vi "Write Serialized Configuration Parameter.vi"(8 "error in (no error)":errorcluster, 10 "Serialized Configuration":string, 11 "RandomNumberLogger in":refnum<class "RandomNumberLogger.lvclass">) -> (0 "error out":errorcluster, 3 "RandomNumberLogger out":refnum<class "RandomNumberLogger.lvclass">)   [LabVIEW 2020, in "RandomNumberLogger.lvlib" / "RandomNumberLogger.lvclass"]
doc: "<b>Write Serialized Configuration Parameter</b>\nThis method writes the serialized configuration data to th class data in the plugin."
uses:
  RandomNumberLogger.lvclass
  C:/Program Files/National Instruments/LabVIEW 2020/vi.lib/FlexLogger/SDK/PluginSDK.lvlibp/PEFClasses/SDK/Processing Element/Processing Element.lvclass
  <vilib>/FlexLogger/SDK/PluginSDK.lvlibp/PEFClasses/SDK/Processing Element/Read Parameters Property.vi
  <vilib>/FlexLogger/SDK/PluginSDK.lvlibp/PEFClasses/SDK/Parameters/SetParameter(String).vi
  <vilib>/FlexLogger/SDK/PluginSDK.lvlibp/PEFClasses/SDK/Processing Element/Write Parameters Property.vi
  <vilib>/FlexLogger/SDK/PluginSDK.lvlibp/PEFClasses/SDK/Parameters/Parameters.lvclass
  RandomNumberLogger.lvclass/RandomNumberLogger.ctl
panel:
  # "#via_ignore"
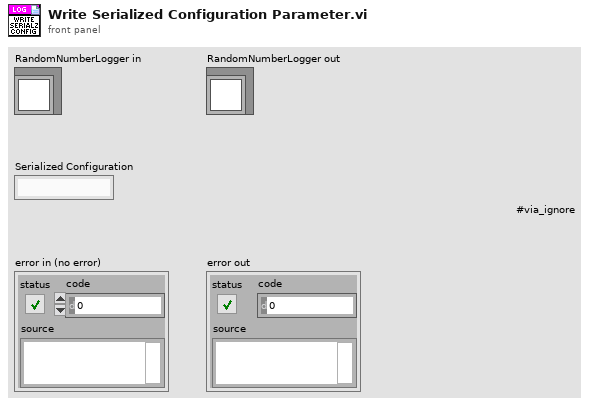
[diagram p1: front panel]
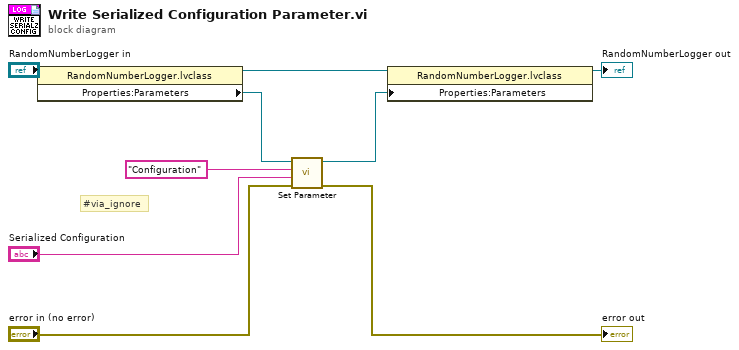
[diagram p0: block diagram]
diagram:
  # "#via_ignore"
  n1 = property on="Property Node" class="RandomNumberLogger.lvclass"(reference="RandomNumberLogger in") -> (reference out=w5:refnum<class "RandomNumberLogger.lvclass">, "Properties:Parameters"=w6:refnum<class "Parameters.lvclass">)  [unwired: 1 in, 1 out]
  n2 = call-poly <vilib>:"Set Parameter.vi"("error in (no error)"="error in (no error)", "Value"="Serialized Configuration", "Name"="Configuration", "Parameters in"=w6) -> ("error out"=→"error out":errorcluster, "Parameters out"=w1:refnum<class "Parameters.lvclass">)  [unwired: 6 in]
  n3 = property on="Property Node" class="RandomNumberLogger.lvclass"(reference=w5, "Properties:Parameters"=w1) -> (reference out=→"RandomNumberLogger out":refnum<class "RandomNumberLogger.lvclass">)  [unwired: 1 in, 1 out]
